vi "Read Transconductance.vi"   [LabVIEW 2019, in "Keithley 2600 Series.lvlib"]
doc: "Performs a source sweep and calculates the transconductance."
uses:
  Keithley 2600 Series.lvlib
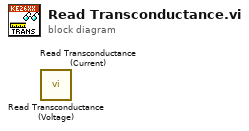
[diagram p0: block diagram]
diagram:
  n1 = call "Read Transconductance (Voltage).vi"() -> ()  [unwired: 11 in, 5 out]
  n2 = call "Read Transconductance (Current).vi"() -> ()  [unwired: 11 in, 5 out]
